vi "f.vi"(0 "2Dピクチャ":picture, 5 "k":i32, 7 "x":dbl, 9 "y":dbl, 11 "error in (no error)":errorcluster caption="エラー入力（エラーなし）") -> (4 "2Dピクチャ":picture, 15 "error out":errorcluster caption="エラー出力")   [LabVIEW 2013]
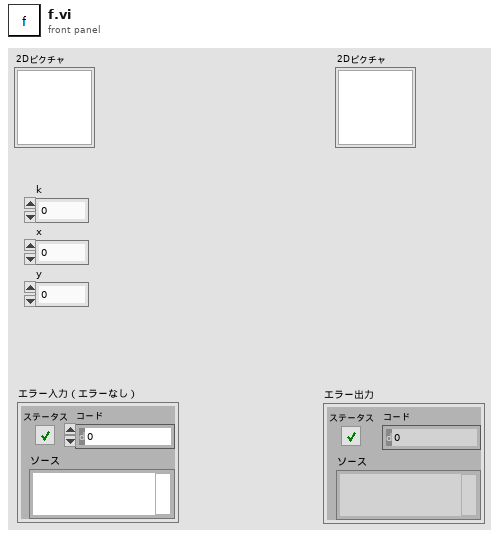
[diagram p1: front panel]
types:
  T1 = enum16{"W1x", "W1y", "W2x", "W2y", "W3x", "W3y", "W4x", "W4y"}
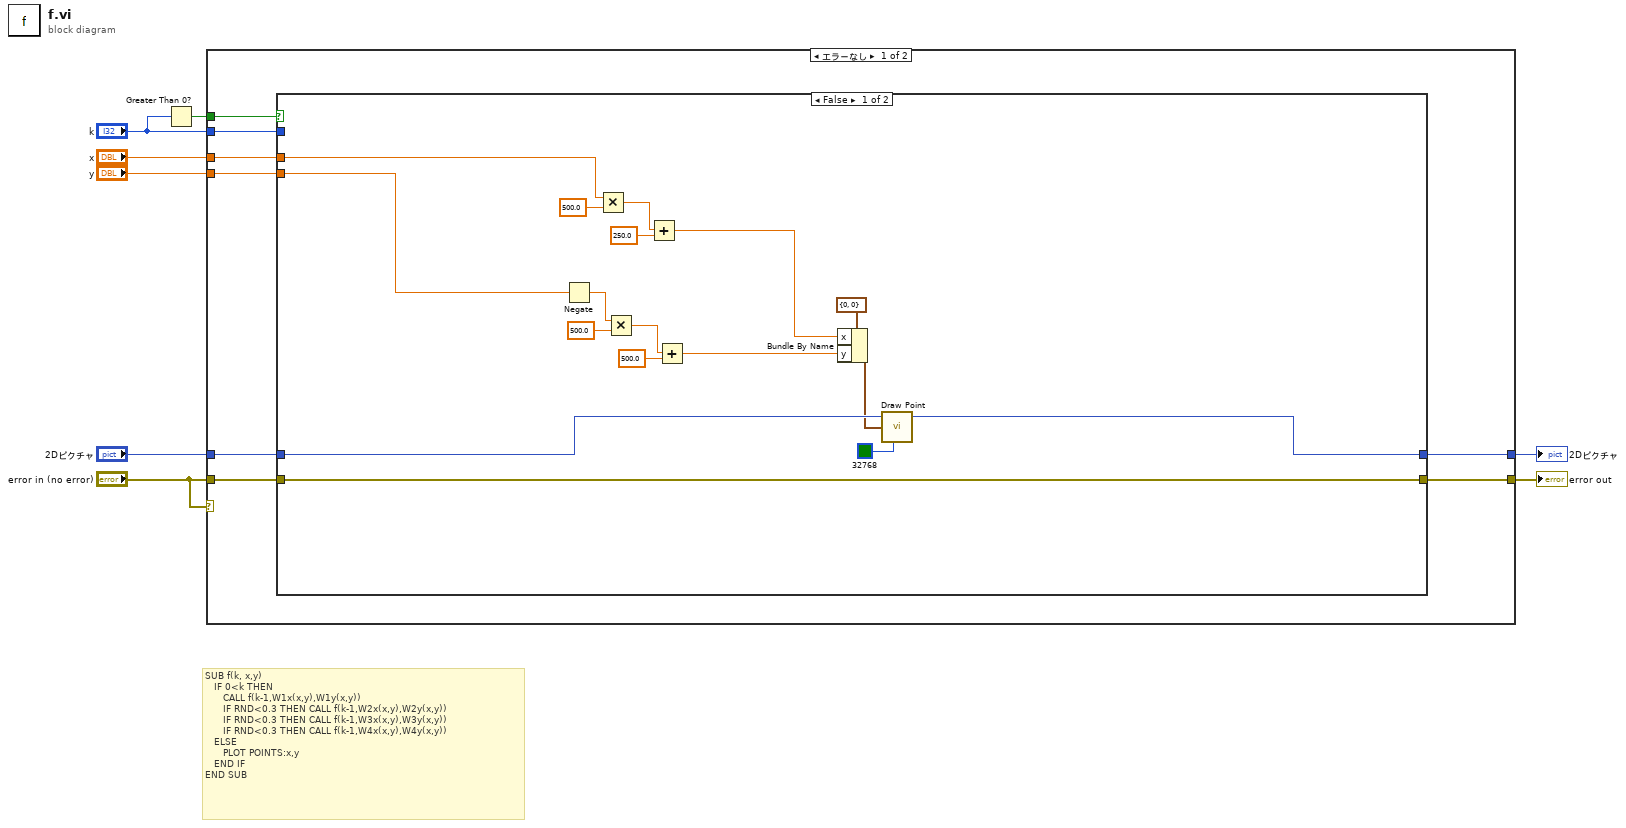
[diagram p0: block diagram]
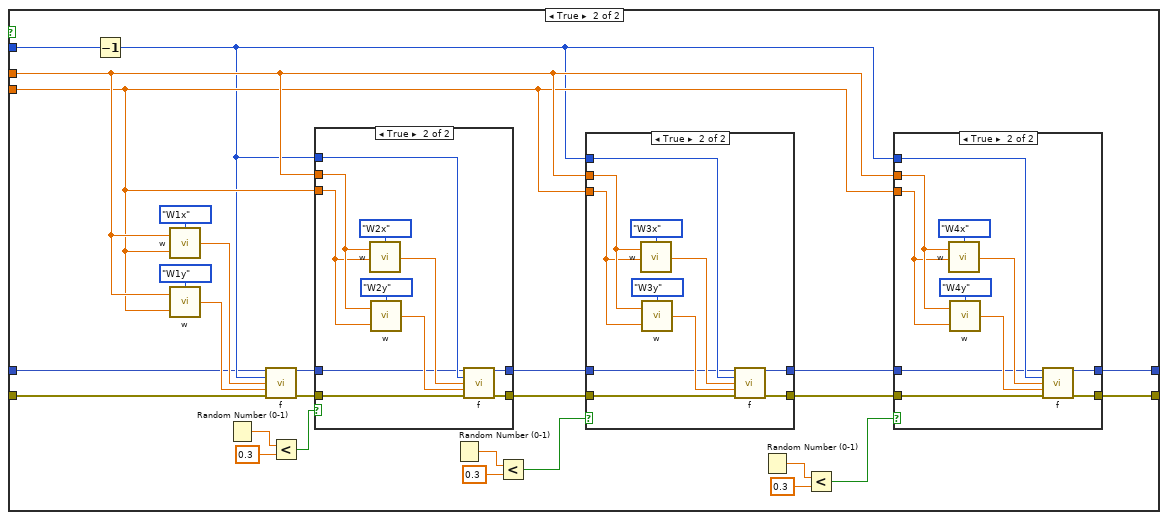
[diagram p2: hidden frame]
diagram:
  # "SUB f(k, x,y)\n   IF 0<k THEN\n      CALL f(k-1,W1x(x,y),W1y(x,y))\n      IF RND<0.3 THEN CALL f(k-1,W2x(x,y),W2y(x,y))\n      IF RND<0.3 THEN CALL f(k-1,W3x(x,y),W3y(x,y))\n      IF RND<0.3 THEN CALL f(k-1,W4x(x,y),W4y(x,y))\n   ELSE\n      PLOT POINTS:x,y\n   END IF\nEND SUB"
  n1 = Greater Than 0?(x="k") -> (x > 0?=w8:bool)
  n2 = case shown="エラーなし" "error in (no error)" {
    tunnel: w8 -> [w16 _]
    tunnel: "k" -> [w15 _]
    tunnel: "x" -> [w14 _]
    tunnel: "y" -> [w13 _]
    tunnel: "error in (no error)" -> [w12 w101]
    tunnel: [w11 w101] -> w4
    tunnel: "2Dピクチャ" -> [w10 w100]
    tunnel: [w9 w100] -> w2
    frame No Error {
      n3 = case shown="FALSE" w16 {
        tunnel: w15 -> [_ w59]
        tunnel: w14 -> [w26 w42]
        tunnel: w13 -> [w23 w41]
        tunnel: w10 -> [w33 w37]
        tunnel: w12 -> [w31 w58]
        tunnel: [w32 w34] -> w9
        tunnel: [w31 w40] -> w11
        frame False {
          n4 = Negate(x=w23) -> (-x=w19:dbl)
          n5 = Multiply(x=w26, y=500.0) -> (x*y=w24:dbl)
          n6 = Multiply(x=w19, y=500.0) -> (x*y=w22:dbl)
          n7 = Add(x=w24, y=250.0) -> (x+y=w17:dbl)
          n8 = Add(x=w22, y=500.0) -> (x+y=w18:dbl)
          n9 = Bundle By Name(cluster=cluster{"x":i16, "y":i16} {"x"=0, "y"=0} ("point(x,y)"), "x"=w17, "y"=w18) -> (w29:cluster{"x":i16, "y":i16})
          n10 = call <vilib>:"Draw Point.vi"("picture"=w33, "point(x,y)"=w29, "color(black)"=u32 32768) -> ("new picture"=w32:picture)  [unwired: 6 in]
        }
        frame True {
          n11 = Decrement(x=w59) -> (x-1=w38:i32)
          n12 = call "w.vi"("関数"=T1."W1x", "y"=w41, "x"=w42) -> ("ret"=w56:dbl)
          n13 = call "w.vi"("関数"=T1."W1y", "y"=w41, "x"=w42) -> ("ret"=w54:dbl)
          n14 = Random Number (0-1)() -> (number: 0 to 1=w53:dbl)
          n15 = call "f.vi"("2Dピクチャ"=w37, "k"=w38, "x"=w56, "y"=w54, "error in (no error)"=w58) -> ("2Dピクチャ"=w39:picture, "error out"=w60:errorcluster)  [unwired: 9 in]
          n16 = Less?(x=w53, y=0.3) -> (x < y?=w51:bool)
          n17 = case shown="TRUE" w51 {
            tunnel: w60 -> [w88 w99]
            tunnel: [w88 w98] -> w50
            tunnel: w42 -> [_ w95]
            tunnel: w41 -> [_ w94]
            tunnel: w38 -> [_ w91]
            tunnel: w39 -> [w87 w90]
            tunnel: [w87 w89] -> w36
            frame False {
            }
            frame True {
              n18 = call "w.vi"("関数"=T1."W2x", "y"=w94, "x"=w95) -> ("ret"=w93:dbl)
              n19 = call "w.vi"("関数"=T1."W2y", "y"=w94, "x"=w95) -> ("ret"=w92:dbl)
              n20 = call "f.vi"("2Dピクチャ"=w90, "k"=w91, "x"=w93, "y"=w92, "error in (no error)"=w99) -> ("2Dピクチャ"=w89:picture, "error out"=w98:errorcluster)  [unwired: 9 in]
            }
          }
          n21 = Random Number (0-1)() -> (number: 0 to 1=w48:dbl)
          n22 = Less?(x=w48, y=0.3) -> (x < y?=w47:bool)
          n23 = case shown="TRUE" w47 {
            tunnel: w50 -> [w75 w86]
            tunnel: [w75 w85] -> w43
            tunnel: w42 -> [_ w82]
            tunnel: w41 -> [_ w81]
            tunnel: w38 -> [_ w78]
            tunnel: w36 -> [w74 w77]
            tunnel: [w74 w76] -> w35
            frame False {
            }
            frame True {
              n24 = call "w.vi"("関数"=T1."W3x", "y"=w81, "x"=w82) -> ("ret"=w80:dbl)
              n25 = call "w.vi"("関数"=T1."W3y", "y"=w81, "x"=w82) -> ("ret"=w79:dbl)
              n26 = call "f.vi"("2Dピクチャ"=w77, "k"=w78, "x"=w80, "y"=w79, "error in (no error)"=w86) -> ("2Dピクチャ"=w76:picture, "error out"=w85:errorcluster)  [unwired: 9 in]
            }
          }
          n27 = Random Number (0-1)() -> (number: 0 to 1=w45:dbl)
          n28 = Less?(x=w45, y=0.3) -> (x < y?=w46:bool)
          n29 = case shown="TRUE" w46 {
            tunnel: w43 -> [w62 w73]
            tunnel: [w62 w72] -> w40
            tunnel: w42 -> [_ w69]
            tunnel: w41 -> [_ w68]
            tunnel: w38 -> [_ w65]
            tunnel: w35 -> [w61 w64]
            tunnel: [w61 w63] -> w34
            frame False {
            }
            frame True {
              n30 = call "w.vi"("関数"=T1."W4x", "y"=w68, "x"=w69) -> ("ret"=w67:dbl)
              n31 = call "w.vi"("関数"=T1."W4y", "y"=w68, "x"=w69) -> ("ret"=w66:dbl)
              n32 = call "f.vi"("2Dピクチャ"=w64, "k"=w65, "x"=w67, "y"=w66, "error in (no error)"=w73) -> ("2Dピクチャ"=w63:picture, "error out"=w72:errorcluster)  [unwired: 9 in]
            }
          }
        }
      }
    }
    frame Error {
    }
  }
  "error out" <- w4
  "2Dピクチャ" <- w2
